vi "MatchRegExSubstrArrayByNumber.vi"(5 "capture index":i32[](array[numeric]), 7 "Options":cluster{"Compile":u32, "Match":u32} {"Match" format="%.0x"; "Compile" format="%.0x"}, 8 "error in":errorcluster, 9 "offset (0)":u64, 10 "search pattern":string, 11 "string":string) -> (0 "error out":errorcluster, 2 "substrings":string[](array[string]), 4 "NextStartOffset":i32, 6 "ContinueMatch?":bool)   [LabVIEW 2021, in "libpcre2-8.lvlib"]
uses:
  libpcre2-8.lvlib
  Pcre2CompileError.vi
  Pcre2ErrorNull.vi
  Pcre2LibError.vi
  Pcre2FnkCallError.vi
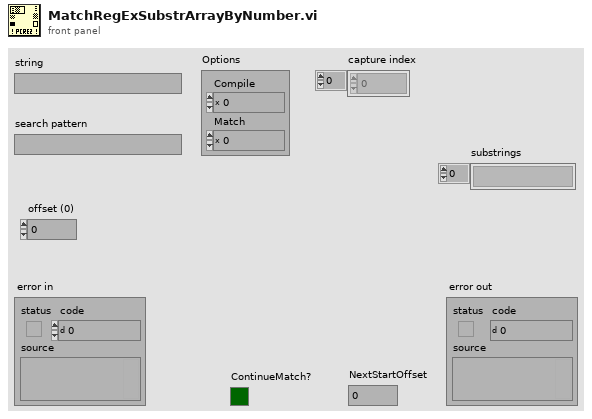
[diagram p1: front panel]
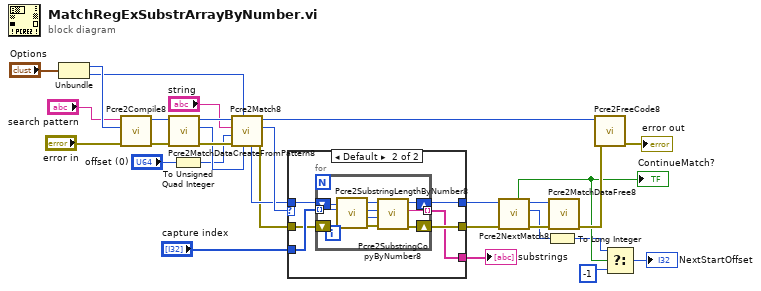
[diagram p0: block diagram]
diagram:
  n1 = Unbundle("Options") -> ("Compile"=w22:u32, "Match"=w21:u32)
  n2 = call "Pcre2Compile8.vi"("error in"="error in", "Options"=w22, "Pattern"="search pattern") -> ("error out"=w28:errorcluster, "pCode"=w27:u64)  [unwired: 7 in]
  n3 = call "Pcre2MatchDataCreateFromPattern8.vi"("error in"=w28, "pCode"=w27) -> ("error out"=w29:errorcluster, "pMatchData"=w20:u64, "pCode"=w30:u64)  [unwired: 7 in]
  n4 = To Unsigned Quad Integer(1:"offset (0)") -> (0:w5:u64)
  n5 = call "Pcre2Match8.vi"("pMatchData"=w20, "Options"=w21, "error in"=w29, "StartOffset"=w5, "Subject"="string", "pCode"=w30) -> ("error out"=w7:errorcluster, "MatchResult"=w9:i32, "pCode"=w26:u64, "pMatchData"=w8:u64)  [unwired: 2 in]
  n6 = case shown="Default" w9 {
    tunnel: w8 -> [w32 w34]
    tunnel: [_ w35] -> w14
    tunnel: [w32 w38] -> w13
    tunnel: "capture index" -> [_ w36]
    tunnel: w7 -> [w31 w33]
    tunnel: [w31 w37] -> w11
    frame ..-1 {
    }
    frame Default {
      n7 = for {
        tunnel: w36 -> [w44] mode=indexing
        tunnel: [w39] -> w35 mode=indexing
        shift-right: [w48] -> w38
        shift-left: w34 -> [w46]
        shift-right: [w47] -> w37
        shift-left: w33 -> [w45]
        n8 = call "Pcre2SubstringLengthByNumber8.vi"("error in"=w45, "Number"=w44, "pMatchData"=w46) -> ("error out"=w43:errorcluster, "Length"=w41:u64, "Number"=w40:i32, "pMatchData"=w42:u64)  [unwired: 5 in]
        n9 = call "Pcre2SubstringCopyByNumber8.vi"("error in"=w43, "Length"=w41, "Number"=w40, "pMatchData"=w42) -> ("error out"=w47:errorcluster, "Substring"=w39:string, "pMatchData"=w48:u64)  [unwired: 5 in]
      }
    }
  }
  "substrings" <- w14
  n10 = call "Pcre2NextMatch8.vi"("error in"=w11, "pMatchData"=w13) -> ("error out"=w10:errorcluster, "NextStartOffset"=w6:u64, "pMatchData"=w12:u64, "ContinueMatch?"=w4:bool)  [unwired: 5 in, 1 out]
  "ContinueMatch?" <- w4
  n11 = To Long Integer(number=w6) -> (32bit integer=w1:i32)
  n12 = call "Pcre2MatchDataFree8.vi"("error in"=w10, "pMatchData"=w12) -> ("error out"=w25:errorcluster)  [unwired: 9 in]
  n13 = call "Pcre2FreeCode8.vi"("error in"=w25, "pCode"=w26) -> ("error out"=→"error out":errorcluster)  [unwired: 9 in]
  n14 = Select(t=w1, s=w4, f=-1) -> (s? t:f=→"NextStartOffset":i32)
